vi "ocpeo.vi"(8 "error in":errorcluster caption="errorIn", 11 "xmlRef":refnum<k20>) -> (0 "error out":errorcluster caption="errorOut", 3 "ocpeo":T1)   [LabVIEW 2017]
uses:
  models/DPF_ocpeo.ctl
  models/DPF_operationMode.ctl
  models/DPF_command.ctl
  models/DPF_pidController.ctl
  models/DPF_engineLimit.ctl
  models/DPF_other.ctl
  <vilib>/xml/Close Reference(Node).vi
  <vilib>/xml/Close Reference(NdList).vi
  <resource>/objmgr/DOMUserDefRef.rc
  <vilib>/xml/NI_XML.lvlib
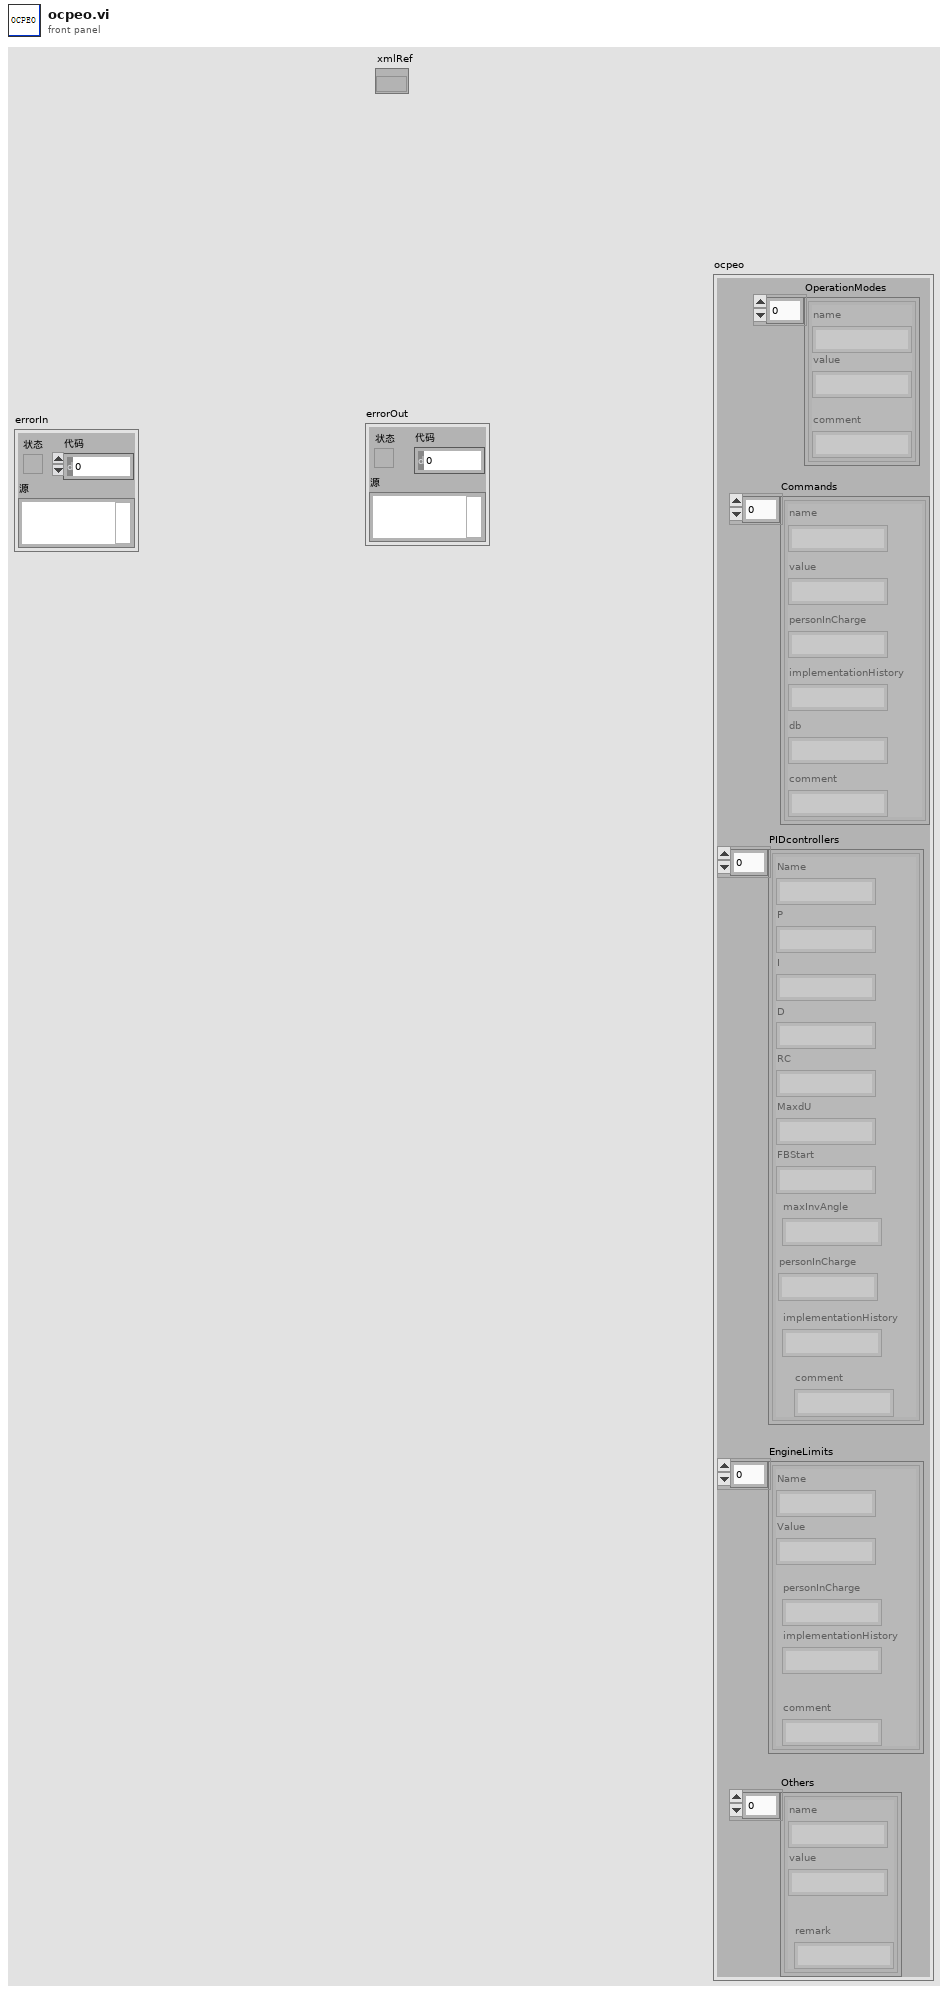
[diagram p1: front panel]
types:
  T1 = typedef "DPF_ocpeo.ctl" = cluster{"OperationModes":T2[], "Commands":T3[], "PIDcontrollers":T4[], "EngineLimits":T5[], "Others":T6[]}
  T2 = typedef "DPF_operationMode.ctl" = cluster{"name":string, "value":string, "comment":string}
  T3 = typedef "DPF_command.ctl" = cluster{"name":string, "value":string, "personInCharge":string, "implementationHistory":string, "db":string, "comment":string}
  T4 = typedef "DPF_pidController.ctl" = cluster{"Name":string, "P":string, "I":string, "D":string, "RC":string, "MaxdU":string, "FBStart":string, "maxInvAngle":string, "personInCharge":string, "implementationHistory":string, "comment":string}
  T5 = typedef "DPF_engineLimit.ctl" = cluster{"Name":string, "Value":string, "personInCharge":string, "implementationHistory":string, "comment":string}
  T6 = typedef "DPF_other.ctl" = cluster{"name":string, "value":string, "remark":string}
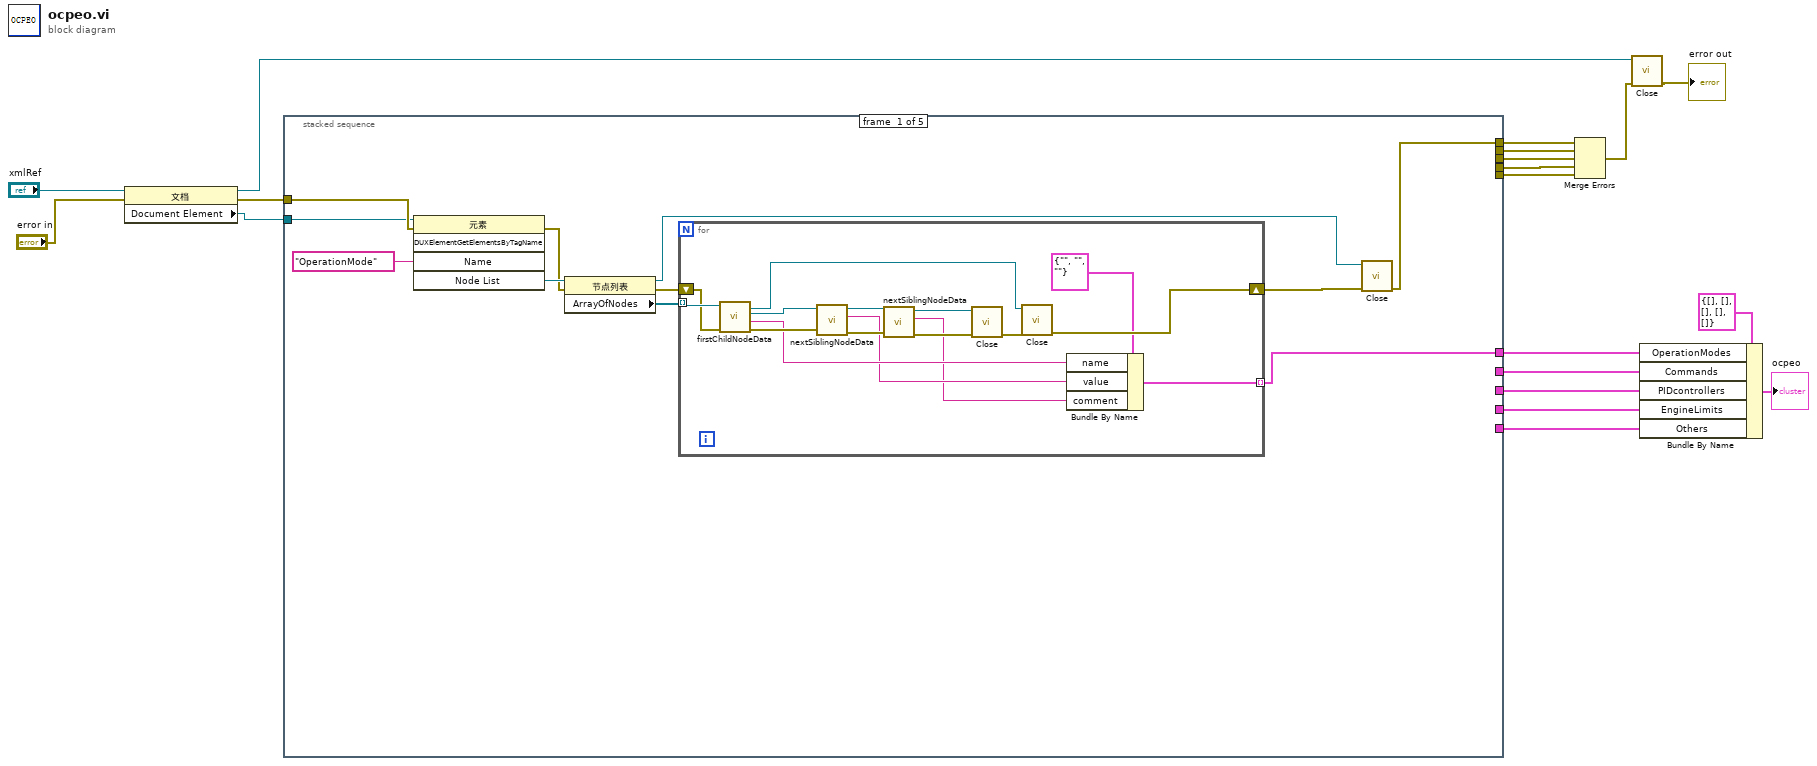
[diagram p0: block diagram]
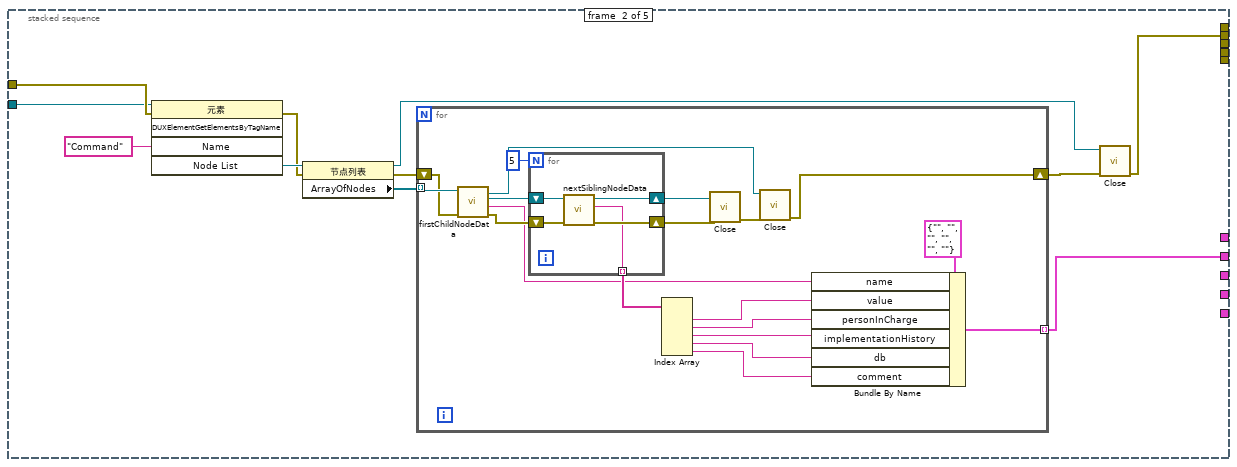
[diagram p2: hidden frame]
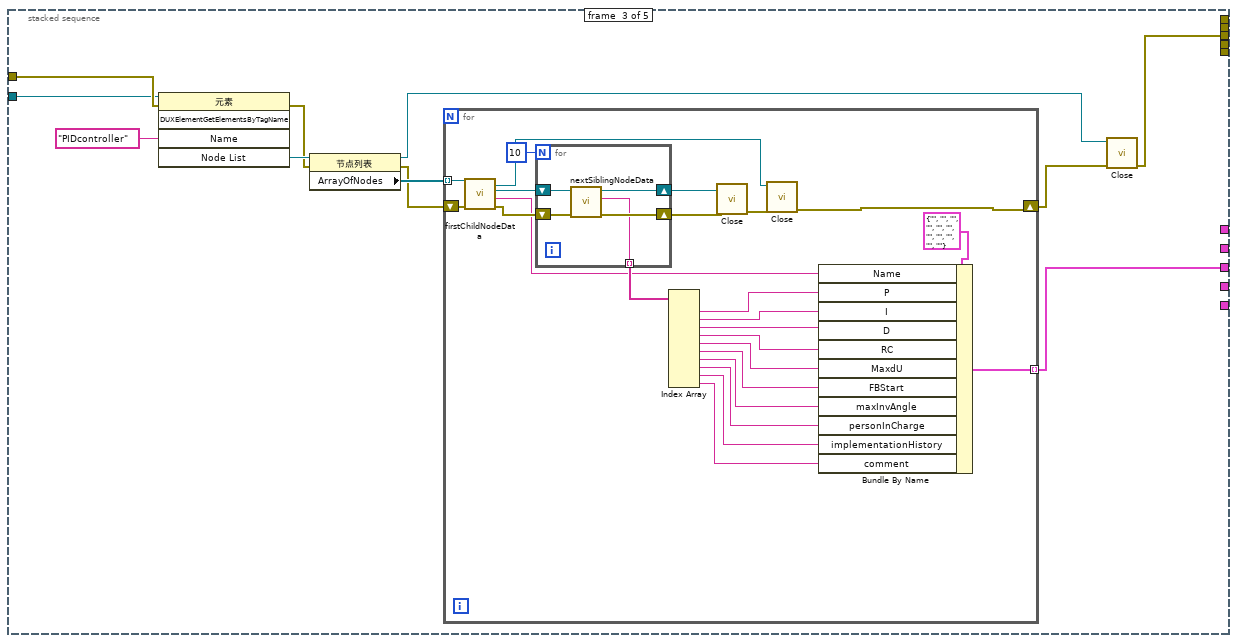
[diagram p3: hidden frame]
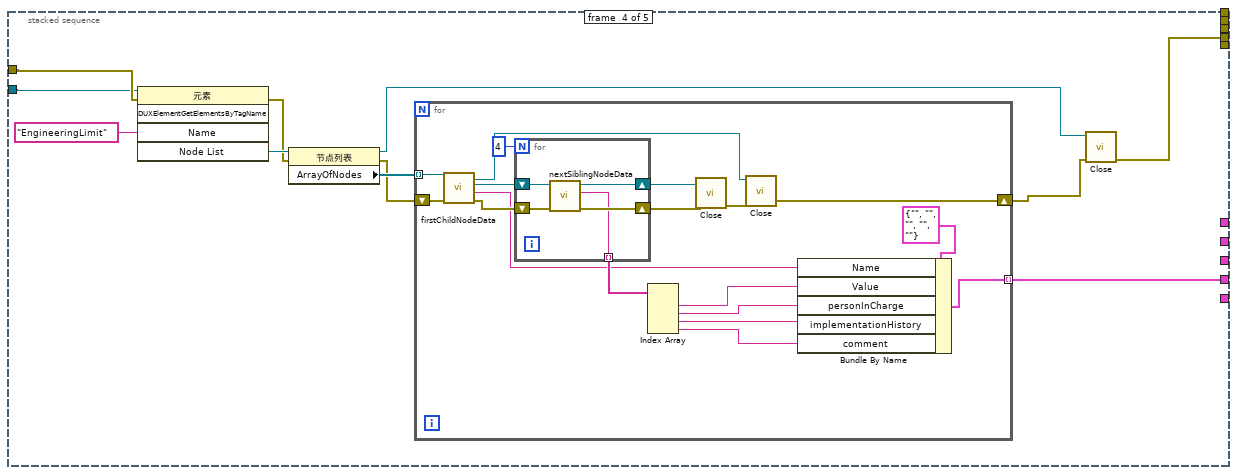
[diagram p4: hidden frame]
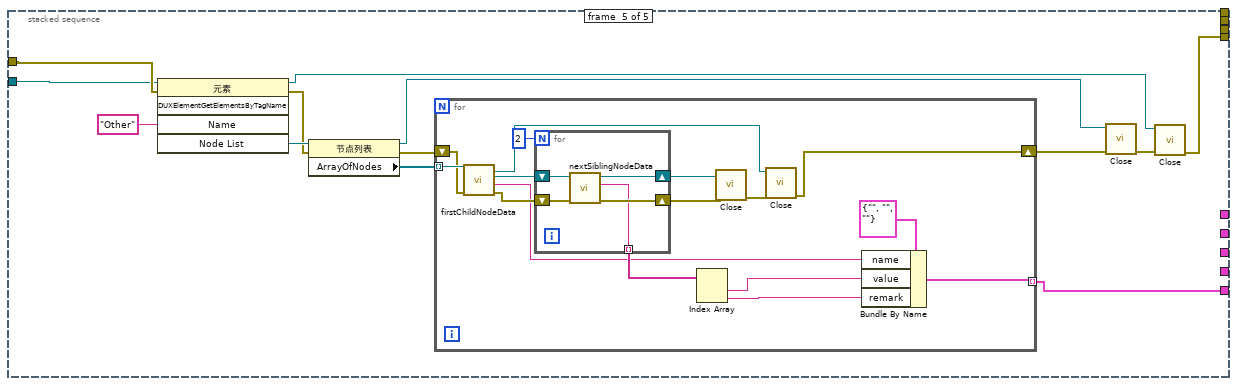
[diagram p5: hidden frame]
diagram:
  n1 = property class="文档"(reference="xmlRef", error in="error in") -> (reference out=w14:refnum<k20>, error out=w19:errorcluster, "Document Element"=w18:refnum<k20>)
  n2 = stacked-sequence {
    tunnel: w19 -> [w29 w50 w88 w128 w162]
    tunnel: w18 -> [w28 w49 w87 w127 w161]
    tunnel: [_ w47 _ _ _] -> w13
    tunnel: [_ _ w82 _ _] -> w12
    tunnel: [_ _ _ _ w157] -> w11
    tunnel: [w21 _ _ _ _] -> w8
    tunnel: [_ w48 _ _ _] -> w7
    tunnel: [_ _ w83 _ _] -> w6
    tunnel: [_ _ _ w123 _] -> w5
    tunnel: [_ _ _ _ w156] -> w4
    tunnel: [_ _ _ w122 _] -> w2
    tunnel: [w20 _ _ _ _] -> w1
    frame #0 {
      n3 = invoke class="元素" method="DUXElementGetElementsByTagName"(reference=w28, error in=w29, "Name"="OperationMode" ("Node Name")) -> (error out=w22:errorcluster, "Node List"=w23:refnum<k20>)  [unwired: 2 in, 3 out]
      n4 = property class="节点列表"(reference=w23, error in=w22) -> (reference out=w25:refnum<k20>, error out=w26:errorcluster, "ArrayOfNodes"=w27:refnum<k20>[])
      n5 = for {
        tunnel: w27 -> [w46] mode=indexing
        shift-right: [w41] -> w24
        shift-left: w26 -> [w40]
        tunnel: [w31] -> w21 mode=indexing
        n6 = call "firstChildNodeData.vi"("error in (no error)"=w40, "parentNode"=w46) -> ("error out"=w44:errorcluster, "data"=w34:string, "childNode"=w45:refnum<k20>, "parentNode"=w42:refnum<k20>)  [unwired: 6 in]
        n7 = call "nextSiblingNodeData.vi"("error in (no error)"=w44, "siblingNode"=w45) -> ("error out"=w38:errorcluster, "data"=w33:string, "childNode"=w39:refnum<k20>)  [unwired: 7 in]
        n8 = call "nextSiblingNodeData.vi"("error in (no error)"=w38, "siblingNode"=w39) -> ("error out"=w36:errorcluster, "data"=w32:string, "childNode"=w37:refnum<k20>)  [unwired: 7 in]
        n9 = call-poly <vilib>:"Close.vi"("error in (no error)"=w36, "node"=w37) -> ("error out"=w43:errorcluster)  [unwired: 7 out]
        n10 = call-poly <vilib>:"Close.vi"("error in (no error)"=w43, "node"=w42) -> ("error out"=w41:errorcluster)  [unwired: 7 out]
        n11 = Bundle By Name(cluster=T2 {"name"="", "value"="", "comment"=""} ("OperationMode"), "name"=w34, "value"=w33, "comment"=w32) -> (w31:T2)
      }
      n12 = call-poly <vilib>:"Close.vi"("error in (no error)"=w24, "node list"=w25) -> ("error out"=w20:errorcluster)  [unwired: 7 out]
    }
    frame #1 {
      n13 = invoke class="元素" method="DUXElementGetElementsByTagName"(reference=w49, error in=w50, "Name"="Command" ("Node Name")) -> (error out=w52:errorcluster, "Node List"=w53:refnum<k20>)  [unwired: 2 in, 3 out]
      n14 = property class="节点列表"(reference=w53, error in=w52) -> (reference out=w55:refnum<k20>, error out=w56:errorcluster, "ArrayOfNodes"=w57:refnum<k20>[])
      n15 = for {
        tunnel: w57 -> [w76] mode=indexing
        shift-right: [w69] -> w54
        shift-left: w56 -> [w58]
        tunnel: [w59] -> w48 mode=indexing
        n16 = call "firstChildNodeData.vi"("error in (no error)"=w58, "parentNode"=w76) -> ("error out"=w74:errorcluster, "data"=w65:string, "childNode"=w75:refnum<k20>, "parentNode"=w70:refnum<k20>)  [unwired: 6 in]
        n17 = for {
          N: 5 -> [_]
          shift-right: [w80] -> w73
          shift-left: w75 -> [w81]
          tunnel: [w77] -> w67 mode=indexing
          shift-right: [w78] -> w72
          shift-left: w74 -> [w79]
          n18 = call "nextSiblingNodeData.vi"("error in (no error)"=w79, "siblingNode"=w81) -> ("error out"=w78:errorcluster, "data"=w77:string, "childNode"=w80:refnum<k20>)  [unwired: 7 in]
        }
        n19 = Index Array(array=w67) -> (element #1=w64:string, element #2=w63:string, element #3=w62:string, element #4=w61:string, element #5=w60:string)  [unwired: 5 in]
        n20 = call-poly <vilib>:"Close.vi"("error in (no error)"=w72, "node"=w73) -> ("error out"=w71:errorcluster)  [unwired: 7 out]
        n21 = call-poly <vilib>:"Close.vi"("error in (no error)"=w71, "node"=w70) -> ("error out"=w69:errorcluster)  [unwired: 7 out]
        n22 = Bundle By Name(cluster=T3 {"name"="", "value"="", "personInCharge"="", "implementationHistory"="", "db"="", "comment"=""} ("Command"), "name"=w65, "value"=w64, "personInCharge"=w63, "implementationHistory"=w62, "db"=w61, "comment"=w60) -> (w59:T3)
      }
      n23 = call-poly <vilib>:"Close.vi"("error in (no error)"=w54, "node list"=w55) -> ("error out"=w47:errorcluster)  [unwired: 7 out]
    }
    frame #2 {
      n24 = invoke class="元素" method="DUXElementGetElementsByTagName"(reference=w87, error in=w88, "Name"="PIDcontroller" ("Node Name")) -> (error out=w90:errorcluster, "Node List"=w91:refnum<k20>)  [unwired: 2 in, 3 out]
      n25 = property class="节点列表"(reference=w91, error in=w90) -> (reference out=w92:refnum<k20>, error out=w85:errorcluster, "ArrayOfNodes"=w86:refnum<k20>[])
      n26 = for {
        tunnel: w86 -> [w101] mode=indexing
        tunnel: [w95] -> w83 mode=indexing
        shift-right: [w93] -> w84
        shift-left: w85 -> [w94]
        n27 = call "firstChildNodeData.vi"("error in (no error)"=w94, "parentNode"=w101) -> ("error out"=w115:errorcluster, "data"=w109:string, "childNode"=w116:refnum<k20>, "parentNode"=w111:refnum<k20>)  [unwired: 6 in]
        n28 = for {
          N: 10 -> [_]
          shift-right: [w120] -> w114
          shift-left: w116 -> [w121]
          tunnel: [w117] -> w110 mode=indexing
          shift-right: [w118] -> w113
          shift-left: w115 -> [w119]
          n29 = call "nextSiblingNodeData.vi"("error in (no error)"=w119, "siblingNode"=w121) -> ("error out"=w118:errorcluster, "data"=w117:string, "childNode"=w120:refnum<k20>)  [unwired: 7 in]
        }
        n30 = Index Array(array=w110) -> (element #1=w108:string, element #2=w107:string, element #3=w106:string, element #4=w105:string, element #5=w104:string, element #6=w100:string, element #7=w99:string, element #8=w98:string, element #9=w97:string, element #10=w96:string)  [unwired: 10 in]
        n31 = call-poly <vilib>:"Close.vi"("error in (no error)"=w113, "node"=w114) -> ("error out"=w112:errorcluster)  [unwired: 7 out]
        n32 = call-poly <vilib>:"Close.vi"("error in (no error)"=w112, "node"=w111) -> ("error out"=w93:errorcluster)  [unwired: 7 out]
        n33 = Bundle By Name(cluster=T4 {"Name"="", "P"="", "I"="", "D"="", "RC"="", "MaxdU"="", "FBStart"="", "maxInvAngle"="", "personInCharge"="", "implementationHistory"="", "comment"=""} ("PIDcontroller"), "Name"=w109, "P"=w108, "I"=w107, "D"=w106, "RC"=w105, "MaxdU"=w104, "FBStart"=w100, "maxInvAngle"=w99, "personInCharge"=w98, "implementationHistory"=w97, "comment"=w96) -> (w95:T4)
      }
      n34 = call-poly <vilib>:"Close.vi"("error in (no error)"=w84, "node list"=w92) -> ("error out"=w82:errorcluster)  [unwired: 7 out]
    }
    frame #3 {
      n35 = invoke class="元素" method="DUXElementGetElementsByTagName"(reference=w127, error in=w128, "Name"="EngineeringLimit" ("Node Name")) -> (error out=w130:errorcluster, "Node List"=w131:refnum<k20>)  [unwired: 2 in, 3 out]
      n36 = property class="节点列表"(reference=w131, error in=w130) -> (reference out=w132:refnum<k20>, error out=w125:errorcluster, "ArrayOfNodes"=w126:refnum<k20>[])
      n37 = for {
        tunnel: w126 -> [w136] mode=indexing
        shift-right: [w134] -> w124
        shift-left: w125 -> [w135]
        tunnel: [w133] -> w123 mode=indexing
        n38 = call "firstChildNodeData.vi"("error in (no error)"=w135, "parentNode"=w136) -> ("error out"=w149:errorcluster, "data"=w143:string, "childNode"=w150:refnum<k20>, "parentNode"=w145:refnum<k20>)  [unwired: 6 in]
        n39 = for {
          N: 4 -> [_]
          shift-right: [w154] -> w148
          shift-left: w150 -> [w155]
          tunnel: [w151] -> w144 mode=indexing
          shift-right: [w152] -> w147
          shift-left: w149 -> [w153]
          n40 = call "nextSiblingNodeData.vi"("error in (no error)"=w153, "siblingNode"=w155) -> ("error out"=w152:errorcluster, "data"=w151:string, "childNode"=w154:refnum<k20>)  [unwired: 7 in]
        }
        n41 = Index Array(array=w144) -> (element #1=w142:string, element #2=w141:string, element #3=w140:string, element #4=w139:string)  [unwired: 4 in]
        n42 = call-poly <vilib>:"Close.vi"("error in (no error)"=w147, "node"=w148) -> ("error out"=w146:errorcluster)  [unwired: 7 out]
        n43 = call-poly <vilib>:"Close.vi"("error in (no error)"=w146, "node"=w145) -> ("error out"=w134:errorcluster)  [unwired: 7 out]
        n44 = Bundle By Name(cluster=T5 {"Name"="", "Value"="", "personInCharge"="", "implementationHistory"="", "comment"=""} ("EngineLimit"), "Name"=w143, "Value"=w142, "personInCharge"=w141, "implementationHistory"=w140, "comment"=w139) -> (w133:T5)
      }
      n45 = call-poly <vilib>:"Close.vi"("error in (no error)"=w124, "node list"=w132) -> ("error out"=w122:errorcluster)  [unwired: 7 out]
    }
    frame #4 {
      n46 = invoke class="元素" method="DUXElementGetElementsByTagName"(reference=w161, error in=w162, "Name"="Other" ("Node Name")) -> (reference out=w166:refnum<k20>, error out=w164:errorcluster, "Node List"=w165:refnum<k20>)  [unwired: 2 in, 2 out]
      n47 = property class="节点列表"(reference=w165, error in=w164) -> (reference out=w168:refnum<k20>, error out=w158:errorcluster, "ArrayOfNodes"=w160:refnum<k20>[])
      n48 = for {
        tunnel: w160 -> [w172] mode=indexing
        tunnel: [w171] -> w156 mode=indexing
        shift-right: [w170] -> w159
        shift-left: w158 -> [w169]
        n49 = call "firstChildNodeData.vi"("error in (no error)"=w169, "parentNode"=w172) -> ("error out"=w183:errorcluster, "data"=w177:string, "childNode"=w184:refnum<k20>, "parentNode"=w179:refnum<k20>)  [unwired: 6 in]
        n50 = for {
          N: 2 -> [_]
          shift-right: [w188] -> w182
          shift-left: w184 -> [w189]
          tunnel: [w185] -> w178 mode=indexing
          shift-right: [w186] -> w181
          shift-left: w183 -> [w187]
          n51 = call "nextSiblingNodeData.vi"("error in (no error)"=w187, "siblingNode"=w189) -> ("error out"=w186:errorcluster, "data"=w185:string, "childNode"=w188:refnum<k20>)  [unwired: 7 in]
        }
        n52 = Index Array(array=w178) -> (element #1=w176:string, element #2=w175:string)  [unwired: 2 in]
        n53 = call-poly <vilib>:"Close.vi"("error in (no error)"=w181, "node"=w182) -> ("error out"=w180:errorcluster)  [unwired: 7 out]
        n54 = call-poly <vilib>:"Close.vi"("error in (no error)"=w180, "node"=w179) -> ("error out"=w170:errorcluster)  [unwired: 7 out]
        n55 = Bundle By Name(cluster=T6 {"name"="", "value"="", "remark"=""} ("Other"), "name"=w177, "value"=w176, "remark"=w175) -> (w171:T6)
      }
      n56 = call-poly <vilib>:"Close.vi"("error in (no error)"=w159, "node list"=w168) -> ("error out"=w167:errorcluster)  [unwired: 7 out]
      n57 = call-poly <vilib>:"Close.vi"("error in (no error)"=w167, "node"=w166) -> ("error out"=w157:errorcluster)  [unwired: 7 out]
    }
  }
  n58 = Merge Errors(w1, w13, w12, w2, w11) -> (w10:errorcluster)
  n59 = call-poly <vilib>:"Close.vi"("error in (no error)"=w10, "node"=w14) -> ("error out"=→"error out":errorcluster)  [unwired: 7 out]
  n60 = Bundle By Name(cluster=T1 {"OperationModes"=[], "Commands"=[], "PIDcontrollers"=[], "EngineLimits"=[], "Others"=[]} ("输入簇"), "OperationModes"=w8, "Commands"=w7, "PIDcontrollers"=w6, "EngineLimits"=w5, "Others"=w4) -> (→"ocpeo":T1)
